vi "DFD Least Pth Norm Design by Newton.vi"(4 "p (128)":i32=128, 5 "pole radius constraint":dbl=0.99 min=0.0, 6 "fs [Hz]":dbl=1.0 format="%.2f", 7 "filter type":T3, 8 "error in (no error)":errorcluster, 9 "group delay":dbl=5.0, 10 "band specs":T1(array[cluster])=[{"frequency point"=[{"frequency"=0.0, "magnitude"=1.0, "weight"=1.0, "phase"=0.0}, {"frequency"=0.2, "magnitude"=1.0, "weight"=1.0, "phase"=0.0}]}, {"frequency point"=[{"frequency"=0.3, "magnitude"=0.0, "weight"=1.0, "phase"=0.0}, {"frequency"=0.5, "magnitude"=0.0, "weight"=1.0, "phase"=0.0}]}] {"frequency point"."weight" format="%.2f"}, 11 "order":cluster{"numerator":i32, "denominator":i32}={"numerator"=5, "denominator"=5}) -> (0 "error out":errorcluster, 2 "pth norm":dbl, 3 "filter out":T4={"mSRate_Fs"=1.0, "mSRate_Version"="2.0", "mSRate_Comments"="", "mSRate_OrgCoef"={"type"=enum."Undefined", "gain"=1.0, "coef a (k)"=[], "coef b (v)"=[]}, "mSRate_CurCoef"={"type"=enum."Undefined", "gain"=1.0, "coef a (k)"=[], "coef b (v)"=[]}, "mSRate_Quantized?"=FALSE, "mSRate_QCoef"={"type"=enum."Undefined", "gain"=1.0, "coef a (k)"=[], "coef b (v)"=[]}, "mSRate_QSettings"=[], "mSRate_Order"=0, "mSRate_Scaling"={"mSRate_ScaleByPowerOf2?"=FALSE, "mSRate_ScaleType"=enum."No Norm"}} {"mSRate_QSettings"."source" items=["Coef a/k"=0, "Coef b/v"=7, "Input"=1, "Output"=2, "Multiplicand"=3, "Product"=4, "Sum"=5, "Delay"=6, "Gain"=8]})   [LabVIEW 2017, in "NI_DigFilterLicensed.lvlib"]
doc: "Designs an infinite impulse response (IIR) or finite impulse response (FIR) filter with a frequency response that matches the response you request in terms of the least pth norm algorithm. You can use either the iterative reweighted least square (IRLS) method or the Newton method that this VI provides to design a filter. You must manually select the polymorphic instance you want to use."
uses:
  <vilib>/addons/Digital Filter Design/NI_DigFilterLicensed.lvlib
  <vilib>/addons/Digital Filter Design/_LpNorm.llb/dfd_Lp Norm Band Spec.ctl
  <vilib>/addons/Digital Filter Design/_Objects.llb/DFD Filter Obj.ctl
  <vilib>/addons/Digital Filter Design/_Objects.llb/DFD Filter Coef.ctl
  <vilib>/addons/Digital Filter Design/_Objects.llb/DFD Filter Structure Type Selector.ctl
  <vilib>/addons/Digital Filter Design/_Objects.llb/dfd_Internal Quantization Settings.ctl
  <vilib>/addons/Digital Filter Design/_Objects.llb/dfd_Internal Quantization Srcs.ctl
  <vilib>/addons/Digital Filter Design/_Objects.llb/DFD Coef Norm Type.ctl
  <vilib>/addons/Digital Filter Design/_LpNorm.llb/dfd_Lp Norm Filter Type.ctl
  <vilib>/addons/Digital Filter Design/_LpNorm.llb/dfd_Lp Norm Design Info.ctl
  <vilib>/addons/Digital Filter Design/NI_DigFilter_Design.lvlib
panel:
  out "IIR Design Info out":T2={"order"={"num"=21, "den"=0}, "p"=2.0, "mag approx?"=FALSE, "radius"=1.0, "freq grid"=[], "d"=[], "weight"=[], "Ha"=[], "Hb"=[], "b & a"=[], "reweight"=[]}
  in  "bands specification":T10 {"magnitude and weight"."frequency point"."weight" format="%.2f"}
  # "phase"
  # "freq"
  # "magnitude"
  # "weight"
  # "frequency"
  # "magnitude"
  # "weight"
  # "phase"
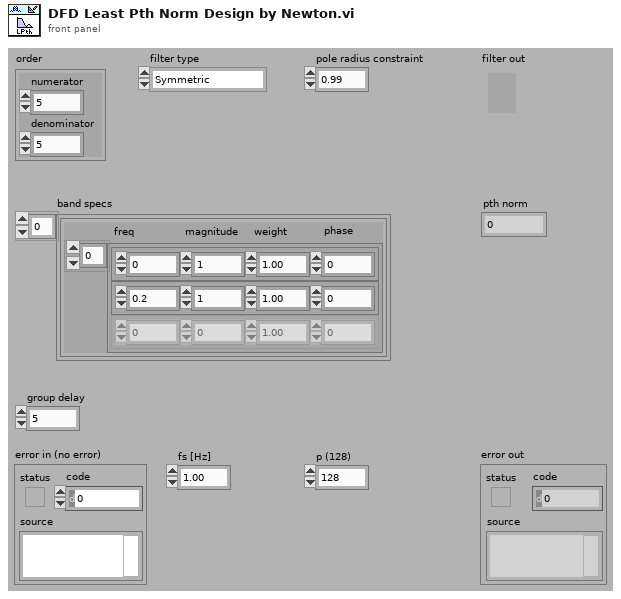
[diagram p1: front panel]
types:
  T1 = cluster{"frequency point":cluster{"frequency":dbl, "magnitude":dbl, "weight":dbl, "phase":dbl}[]}[]
  T2 = typedef "dfd_Lp Norm Design Info.ctl" = cluster{"order":cluster{"num":i32, "den":i32}, "p":dbl, "mag approx?":bool, "radius":dbl, "freq grid":dbl[], "d":cdb[], "weight":dbl[], "Ha":cdb[][], "Hb":cdb[][], "b & a":dbl[], "reweight":dbl[]}
  T3 = typedef "NI_DigFilterLicensed.lvlib/dfd_Lp Norm Filter Type.ctl" = enum16{"Symmetric", "Antisymmetric", "Differentiator", "Hilbert", "Minimum Phase", "Maximum Phase"}
  T4 = typedef "NI_DigFilterLicensed.lvlib/DFD Filter Obj.ctl" = cluster{"mSRate_Fs":dbl, "mSRate_Version":string, "mSRate_Comments":string, "mSRate_OrgCoef":T5, "mSRate_CurCoef":T5, "mSRate_Quantized?":bool, "mSRate_QCoef":T5, "mSRate_QSettings":T7[], "mSRate_Order":i32, "mSRate_Scaling":cluster{"mSRate_ScaleByPowerOf2?":bool, "mSRate_ScaleType":T9}}
  T5 = typedef "NI_DigFilterLicensed.lvlib/DFD Filter Coef.ctl" = cluster{"type":T6, "gain":dbl, "coef a (k)":dbl[], "coef b (v)":dbl[]}
  T6 = typedef "NI_DigFilterLicensed.lvlib/DFD Filter Structure Type Selector.ctl" = enum16{"Undefined", "FIR Direct Form", "FIR Direct Form Transposed", "FIR Symmetric", "FIR Antisymmetric", "IIR Direct Form I", "IIR Direct Form I Transposed", "IIR Direct Form II", "IIR Direct Form II Transposed", "IIR Cascaded Second Order Sections Form I", "IIR Cascaded Second Order Sections Form I Transposed", "IIR Cascaded Second Order Sections Form II", "IIR Cascaded Second Order Sections Form II Transposed", "Lattice Allpass (basic sections)", "Lattice Allpass (one multiplier sections)", "Lattice Allpass (normalized sections)", "Lattice AR (basic sections)", "Lattice AR (one multiplier sections)", "Lattice AR (normalized sections)", "Lattice MA (minimum phase)", "Lattice MA (maximum phase)", "Lattice ARMA (basic sections)", "Lattice ARMA (one multiplier sections)", "Lattice ARMA (normalized sections)"}
  T7 = typedef "NI_DigFilterLicensed.lvlib/dfd_Internal Quantization Settings.ctl" = cluster{"source":T8, "wl":i16, "iwl":i16, "overflow mode":enum16{"Saturation", "Wrap"}, "rounding mode":enum16{"Nearest", "Truncation"}, "signed?":bool}
  T8 = typedef "NI_DigFilterLicensed.lvlib/dfd_Internal Quantization Srcs.ctl" = u16
  T9 = typedef "NI_DigFilterLicensed.lvlib/DFD Coef Norm Type.ctl" = enum16{"No Norm", "Time Domain 1-Norm", "Time Domain 2-Norm", "Time Domain Inf-Norm"}
  T10 = typedef "dfd_Lp Norm Band Spec.ctl" = cluster{"magnitude and weight":cluster{"frequency point":cluster{"frequency":dbl, "magnitude":dbl, "weight":dbl, "phase":dbl}[]}[], "group delay":dbl}
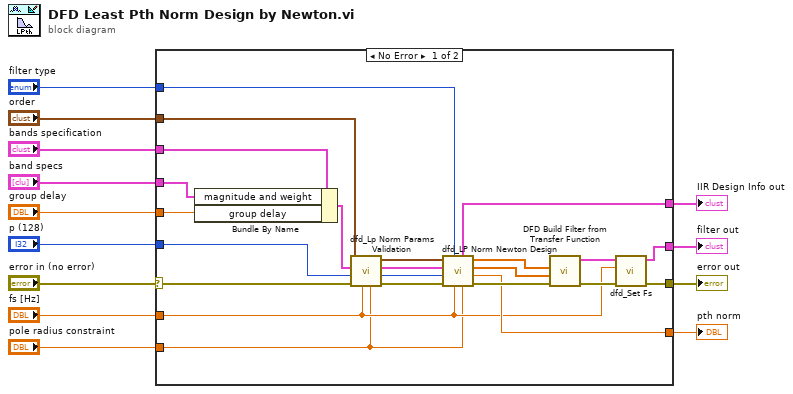
[diagram p0: block diagram]
diagram:
  n1 = case shown="No Error" "error in (no error)" {
    selector: "error in (no error)" -> [w14 w37]
    tunnel: [w32 _] -> w13
    tunnel: [w30 _] -> w12
    tunnel: "filter type" -> [w29 _]
    tunnel: [w28 _] -> w10
    tunnel: "p (128)" -> [w26 _]
    tunnel: "order" -> [w23 _]
    tunnel: "fs [Hz]" -> [w22 _]
    tunnel: "pole radius constraint" -> [w20 _]
    tunnel: "bands specification" -> [w18 _]
    tunnel: "band specs" -> [w17 _]
    tunnel: "group delay" -> [w16 _]
    tunnel: [w15 w37] -> w2
    frame No Error {
      n2 = Bundle By Name(cluster=w18, "magnitude and weight"=w17, "group delay"=w16) -> (w19:T10)
      n3 = call <vilib>:"dfd_Lp Norm Params Validation.vi"("max pole radius"=w20, "fs [Hz]"=w22, "error in (no error)"=w14, "p"=w26, "bands spec"=w19, "order"=w23) -> ("error out"=w21:errorcluster, "p out"=w25:i32, "dup bands spec"=w27:T10, "dup order"=w24:cluster{"num":i32, "den":i32})  [unwired: 2 out]
      n4 = call <vilib>:"dfd_LP Norm Newton Design.vi"("radius constraint?"=w20, "sampling frequency"=w22, "filter type"=w29, "error in (no error)"=w21, "p"=w25, "band specification"=w27, "order"=w24) -> ("error out"=w31:errorcluster, "function value"=w30:dbl, "denominator"=w35:dbl[], "numerator"=w36:dbl[], "dup IIR Design Info"=w28:T2)
      n5 = call <vilib>:"DFD Build Filter from Transfer Function.vi"("error in (no error)"=w31, "denominator"=w35, "numerator"=w36) -> ("error out"=w33:errorcluster, "filter out"=w34:T4)  [unwired: 1 in, 6 out]
      n6 = call <vilib>:"dfd_Set Fs.vi"("error in (no error)"=w33, "fs [Hz]"=w22, "filter in"=w34) -> ("error out"=w15:errorcluster, "filter out"=w32:T4)  [unwired: 7 out]
    }
    frame Error {
    }
  }
  "filter out" <- w13
  "error out" <- w2
  "pth norm" <- w12
  "IIR Design Info out" <- w10
